vi "CallC.vi"(8 "error in (no error)":errorcluster, 11 "stripped path":path) -> (0 "error out":errorcluster)   [LabVIEW 2020]
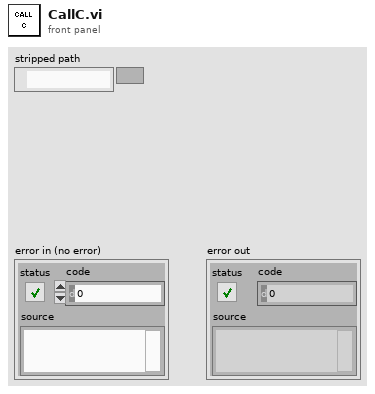
[diagram p1: front panel]
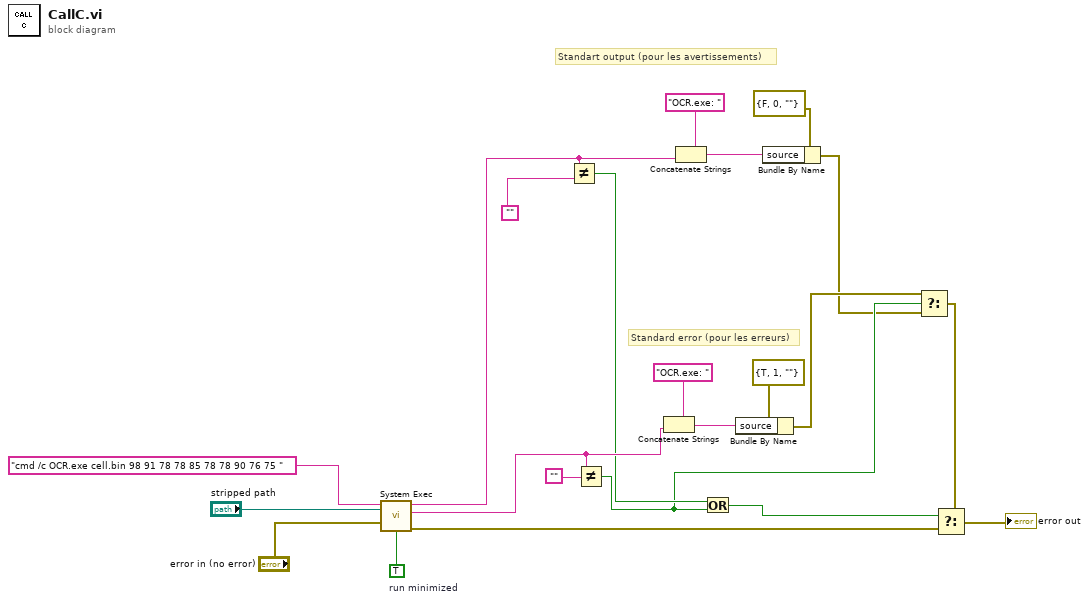
[diagram p0: block diagram]
diagram:
  w22 = TRUE  # run minimized
  # "Standard error (pour les erreurs)"
  # "Standart output (pour les avertissements)"
  n1 = call <vilib>:"System Exec.vi"("run minimized? (F)"=w22, "error in (no error)"="error in (no error)", "working directory"="stripped path", "command line"="cmd /c OCR.exe cell.bin 98 91 78 78 85 78 78 90 76 75 ") -> ("error out"=w18:errorcluster, "standard error"=w9:string, "standard output"=w7:string)  [unwired: 4 in, 1 out]
  n2 = Not Equal?(x=w7, y="") -> (x != y?=w5:bool)
  n3 = Not Equal?(x="", y=w9) -> (x != y?=w4:bool)
  n4 = Concatenate Strings("OCR.exe: ", w9) -> (w14:string)
  n5 = Concatenate Strings("OCR.exe: ", w7) -> (w6:string)
  n6 = Or(x=w5, y=w4) -> (x .or. y?=w12:bool)
  n7 = Bundle By Name(cluster=errorcluster {"status"=TRUE, "code"=1, "source"=""}, "source"=w14) -> (w3:errorcluster)
  n8 = Bundle By Name(cluster=errorcluster {"status"=FALSE, "code"=0, "source"=""}, "source"=w6) -> (w2:errorcluster)
  n9 = Select(t=w3, s=w4, f=w2) -> (s? t:f=w1:errorcluster)
  n10 = Select(t=w1, s=w12, f=w18) -> (s? t:f=→"error out":errorcluster)
